vi "Finish.vi"   [LabVIEW 2016]
doc: "This VI is called just before exiting. It is expected to close I/O refnum, save collected data, etc."
uses:
  <vilib>/Rock Robotics/WPI/Utilities/WPI_GetSetVariantRefNum.vi
types:
  T1 = typedef "WPI_EncoderDevRef.ctl" = cluster{"DevStatus":errorcluster, "EncoderIndex":T2, "CounterIndex":T3, "DistancePerCount":dbl, "Decoding Type":T4}
  T2 = typedef "FPGA_EncoderIdx.ctl" = enum8{"Enc 0", "Enc 1", "Enc 2", "Enc 3", "Enc 4", "Enc 5", "Enc 6", "Enc 7", "Invalid"}
  T3 = typedef "FPGA_CounterCtrSystemIndex.ctl" = enum8{"Ctr 0", "Ctr 1", "Ctr 2", "Ctr 3", "Ctr 4", "Ctr 5", "Ctr 6", "Ctr 7", "Invalid"}
  T4 = typedef "WPI_EncoderType.ctl" = enum16{"1x", "2x", "4x"}
  T5 = typedef "WPI_DigitalOutputDevRef.ctl" = cluster{"DIO Channel":T6, "DevStatus":errorcluster}
  T6 = typedef "FPGA_DIOChannel.ctl" = enum8{"DIO 0", "DIO 1", "DIO 2", "DIO 3", "DIO 4", "DIO 5", "DIO 6", "DIO 7", "DIO 8", "DIO 9", "DIO MXP 0", "DIO MXP 1", "DIO MXP 2", "DIO MXP 3", "DIO MXP 4", "DIO MXP 5", "DIO MXP 6", "DIO MXP 7", "DIO MXP 8", "DIO MXP 9", "DIO MXP 10", "DIO MXP 11", "DIO MXP 12", "DIO MXP 13", "DIO MXP 14", "DIO MXP 15", "SPI Port CS1", "SPI Port CS2", "SPI Port CS3", "SPI Port MISO", "SPI Port MOSI", "Invalid"}
  T7 = typedef "WPI_RobotDriveDevRef.ctl" = cluster{"DevStatus":errorcluster, "Motors[]":T8[], "Square Inputs":bool, "Max Output":dbl}
  T8 = typedef "WPI_MotorControlDeviceRef.ctl" = cluster{"DeviceStatus":errorcluster, "Type":T9, "PWM":cluster{"PWM Channel":T10, "DeadBand":T11}, "CAN":cluster{"Device Number":u8, "SetOutput VI Ref":variant, "GetOutput VI Ref":variant, "Enable VI Ref":variant, "Disable VI Ref":variant, "Data":variant}, "Invert":bool}
  T9 = typedef "WPI_MotorControlType.ctl" = enum16{"PWM", "CAN"}
  T10 = typedef "FPGA_DIOPWMChannel.ctl" = enum8{"PWM 0", "PWM 1", "PWM 2", "PWM 3", "PWM 4", "PWM 5", "PWM 6", "PWM 7", "PWM 8", "PWM 9", "PWM MXP 0", "PWM MXP 1", "PWM MXP 2", "PWM MXP 3", "PWM MXP 4", "PWM MXP 5", "PWM MXP 6", "PWM MXP 7", "PWM MXP 8", "PWM MXP 9", "Invalid"}
  T11 = typedef "WPI_PWMDeadband.ctl" = cluster{"Name":string, "maxPositivePwm":i32, "minPositivePwm":i32, "centerPwm":i32, "maxNegativePwm":i32, "minNegativePwm":i32, "angularRange":u16}
  T12 = typedef "WPI_JoystickDevRef.ctl" = cluster{"Device":T13}
  T13 = typedef "WPI_JoystickDeviceEnum.ctl" = enum16{"USB 0", "USB 1", "USB 2", "USB 3", "USB 4", "USB 5"}
  T14 = typedef "WPI_SolenoidDevRef.ctl" = cluster{"DevStatus":errorcluster, "Pneumatics Control Module":u8, "Forward Solenoid Channel":T15, "Reverse Solenoid Channel":T15}
  T15 = typedef "WPI_SolenoidChannel.ctl" = enum8{"Solenoid 0", "Solenoid 1", "Solenoid 2", "Solenoid 3", "Solenoid 4", "Solenoid 5", "Solenoid 6", "Solenoid 7", "Invalid"}
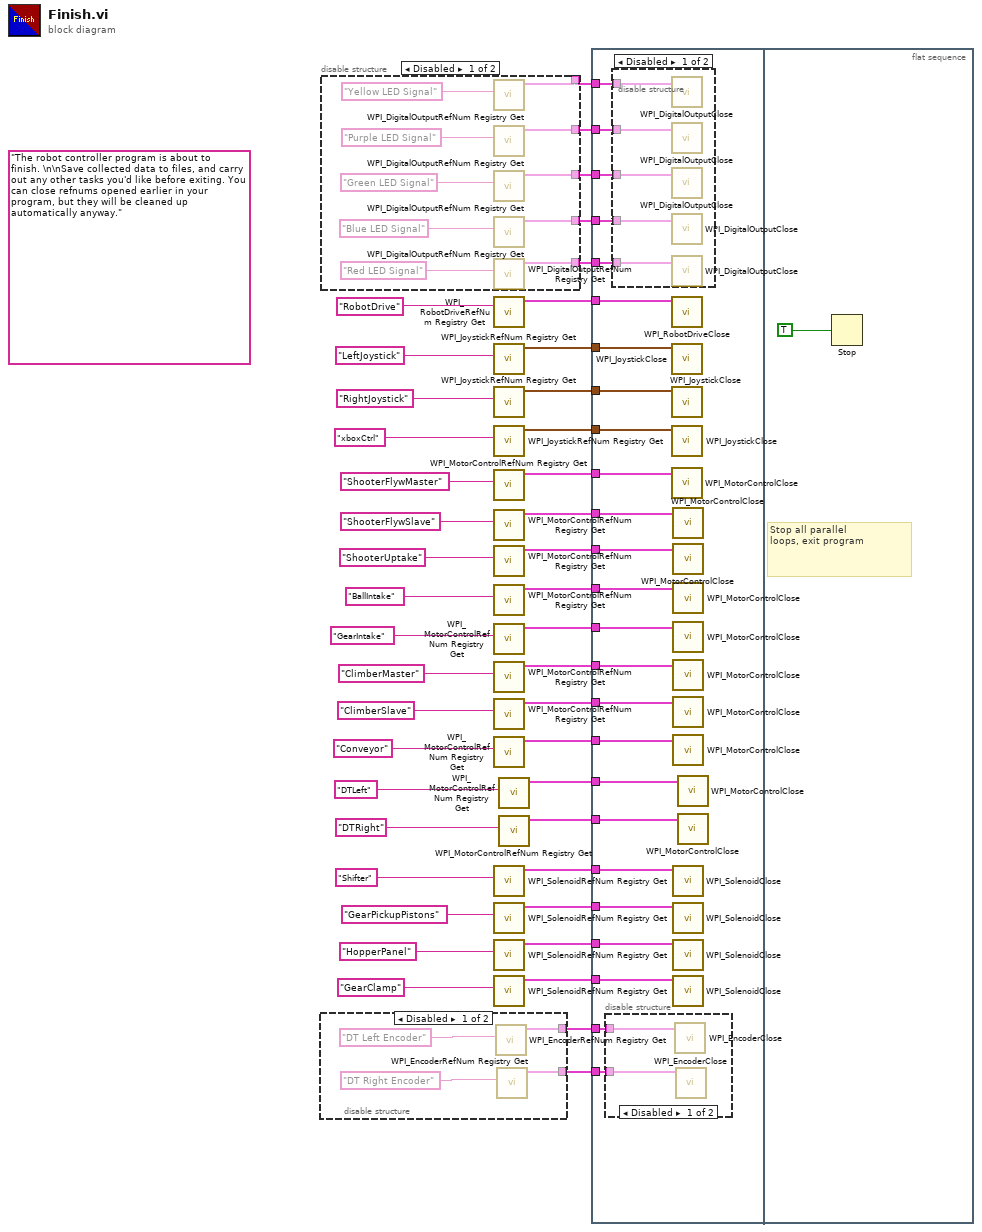
[diagram p0: block diagram]
diagram:
  (unwired) "The robot controller program is about to finish. \n\nSave collected data to files, and carry out any other tasks you'd like before exiting. You can close refnums opened earlier in your program, but they will be cleaned up automatically anyway."
  n1 = disable-structure shown="Disabled" {
    disable-tunnel: [w45 _] -> w6
    disable-tunnel: [w44 _] -> w5
    frame Disabled {
      n2 = call <vilib>:"WPI_EncoderRefNum Registry Get.vi"("refnum name"="DT Left Encoder") -> ("EncoderDevRef"=w45:T1)  [unwired: 9 in, 1 out]
      n3 = call <vilib>:"WPI_EncoderRefNum Registry Get.vi"("refnum name"="DT Right Encoder") -> ("EncoderDevRef"=w44:T1)  [unwired: 9 in, 1 out]
    }
    frame Enabled {
    }
  }
  n4 = disable-structure shown="Disabled" {
    disable-tunnel: [w57 _] -> w11
    disable-tunnel: [w56 _] -> w10
    disable-tunnel: [w55 _] -> w9
    disable-tunnel: [w54 _] -> w8
    disable-tunnel: [w53 _] -> w7
    frame Disabled {
      n5 = call <vilib>:"WPI_DigitalOutputRefNum Registry Get.vi"("refnum name"="Yellow LED Signal") -> ("DigitalOutputDevRef"=w53:T5)  [unwired: 9 in, 1 out]
      n6 = call <vilib>:"WPI_DigitalOutputRefNum Registry Get.vi"("refnum name"="Purple LED Signal") -> ("DigitalOutputDevRef"=w54:T5)  [unwired: 9 in, 1 out]
      n7 = call <vilib>:"WPI_DigitalOutputRefNum Registry Get.vi"("refnum name"="Green LED Signal") -> ("DigitalOutputDevRef"=w55:T5)  [unwired: 9 in, 1 out]
      n8 = call <vilib>:"WPI_DigitalOutputRefNum Registry Get.vi"("refnum name"="Blue LED Signal") -> ("DigitalOutputDevRef"=w56:T5)  [unwired: 9 in, 1 out]
      n9 = call <vilib>:"WPI_DigitalOutputRefNum Registry Get.vi"("refnum name"="Red LED Signal") -> ("DigitalOutputDevRef"=w57:T5)  [unwired: 9 in, 1 out]
    }
    frame Enabled {
    }
  }
  n10 = call <vilib>:"WPI_RobotDriveRefNum Registry Get.vi"("refnum name"="RobotDrive") -> ("RobotDriveDevRef"=w41:T7)  [unwired: 1 in, 9 out]
  n11 = call <vilib>:"WPI_JoystickRefNum Registry Get.vi"("refnum name"="LeftJoystick") -> ("JoystickDevRef"=w40:T12)  [unwired: 1 in, 9 out]
  n12 = call <vilib>:"WPI_JoystickRefNum Registry Get.vi"("refnum name"="RightJoystick") -> ("JoystickDevRef"=w39:T12)  [unwired: 1 in, 9 out]
  n13 = call <vilib>:"WPI_JoystickRefNum Registry Get.vi"("refnum name"="xboxCtrl") -> ("JoystickDevRef"=w36:T12)  [unwired: 1 in, 9 out]
  n14 = call <vilib>:"WPI_MotorControlRefNum Registry Get.vi"("refnum name"="ShooterFlywMaster") -> ("MotorControlDevRef"=w35:T8)  [unwired: 9 in, 1 out]
  n15 = call <vilib>:"WPI_MotorControlRefNum Registry Get.vi"("refnum name"="ShooterFlywSlave") -> ("MotorControlDevRef"=w32:T8)  [unwired: 9 in, 1 out]
  n16 = call <vilib>:"WPI_MotorControlRefNum Registry Get.vi"("refnum name"="ShooterUptake") -> ("MotorControlDevRef"=w31:T8)  [unwired: 9 in, 1 out]
  n17 = call <vilib>:"WPI_MotorControlRefNum Registry Get.vi"("refnum name"="BallIntake") -> ("MotorControlDevRef"=w28:T8)  [unwired: 9 in, 1 out]
  n18 = call <vilib>:"WPI_MotorControlRefNum Registry Get.vi"("refnum name"="GearIntake") -> ("MotorControlDevRef"=w27:T8)  [unwired: 9 in, 1 out]
  n19 = call <vilib>:"WPI_MotorControlRefNum Registry Get.vi"("refnum name"="ClimberMaster") -> ("MotorControlDevRef"=w24:T8)  [unwired: 9 in, 1 out]
  n20 = call <vilib>:"WPI_MotorControlRefNum Registry Get.vi"("refnum name"="ClimberSlave") -> ("MotorControlDevRef"=w23:T8)  [unwired: 9 in, 1 out]
  n21 = call <vilib>:"WPI_MotorControlRefNum Registry Get.vi"("refnum name"="Conveyor") -> ("MotorControlDevRef"=w20:T8)  [unwired: 9 in, 1 out]
  n22 = call <vilib>:"WPI_SolenoidRefNum Registry Get.vi"("refnum name"="Shifter") -> ("SolenoidDevRef"=w19:T14)  [unwired: 9 in, 1 out]
  n23 = call <vilib>:"WPI_SolenoidRefNum Registry Get.vi"("refnum name"="GearPickupPistons") -> ("SolenoidDevRef"=w16:T14)  [unwired: 9 in, 1 out]
  n24 = call <vilib>:"WPI_SolenoidRefNum Registry Get.vi"("refnum name"="HopperPanel") -> ("SolenoidDevRef"=w15:T14)  [unwired: 9 in, 1 out]
  n25 = call <vilib>:"WPI_SolenoidRefNum Registry Get.vi"("refnum name"="GearClamp") -> ("SolenoidDevRef"=w12:T14)  [unwired: 9 in, 1 out]
  n26 = call <vilib>:"WPI_MotorControlRefNum Registry Get.vi"("refnum name"="DTLeft") -> ("MotorControlDevRef"=w1:T8)  [unwired: 9 in, 1 out]
  n27 = call <vilib>:"WPI_MotorControlRefNum Registry Get.vi"("refnum name"="DTRight") -> ("MotorControlDevRef"=w4:T8)  [unwired: 9 in, 1 out]
  n28 = flat-sequence {
    tunnel: w41 -> [w82]
    tunnel: w40 -> [w81]
    tunnel: w39 -> [w80]
    tunnel: w36 -> [w79]
    tunnel: w35 -> [w78]
    tunnel: w32 -> [w77]
    tunnel: w31 -> [w76]
    tunnel: w28 -> [w75]
    tunnel: w27 -> [w74]
    tunnel: w24 -> [w73]
    tunnel: w23 -> [w72]
    tunnel: w20 -> [w71]
    tunnel: w19 -> [w70]
    tunnel: w16 -> [w69]
    tunnel: w15 -> [w68]
    tunnel: w12 -> [w67]
    tunnel: w11 -> [w66]
    tunnel: w10 -> [w65]
    tunnel: w9 -> [w64]
    tunnel: w8 -> [w63]
    tunnel: w7 -> [w62]
    tunnel: w6 -> [w61]
    tunnel: w5 -> [w60]
    tunnel: w1 -> [w58]
    tunnel: w4 -> [w59]
    frame #0 {
      n29 = disable-structure shown="Disabled" {
        disable-tunnel: w61 -> [w89 _]
        disable-tunnel: w60 -> [w88 _]
        frame Disabled {
          n30 = call <vilib>:"WPI_EncoderClose.vi"("EncoderDevRef"=w89) -> ()  [unwired: 10 in, 1 out]
          n31 = call <vilib>:"WPI_EncoderClose.vi"("EncoderDevRef"=w88) -> ()  [unwired: 10 in, 1 out]
        }
        frame Enabled {
        }
      }
      n32 = disable-structure shown="Disabled" {
        disable-tunnel: w66 -> [w87 _]
        disable-tunnel: w65 -> [w86 _]
        disable-tunnel: w64 -> [w85 _]
        disable-tunnel: w63 -> [w84 _]
        disable-tunnel: w62 -> [w83 _]
        frame Disabled {
          n33 = call <vilib>:"WPI_DigitalOutputClose.vi"("DigitalOutputDevRef"=w83) -> ()  [unwired: 10 in, 1 out]
          n34 = call <vilib>:"WPI_DigitalOutputClose.vi"("DigitalOutputDevRef"=w84) -> ()  [unwired: 10 in, 1 out]
          n35 = call <vilib>:"WPI_DigitalOutputClose.vi"("DigitalOutputDevRef"=w85) -> ()  [unwired: 10 in, 1 out]
          n36 = call <vilib>:"WPI_DigitalOutputClose.vi"("DigitalOutputDevRef"=w86) -> ()  [unwired: 10 in, 1 out]
          n37 = call <vilib>:"WPI_DigitalOutputClose.vi"("DigitalOutputDevRef"=w87) -> ()  [unwired: 10 in, 1 out]
        }
        frame Enabled {
        }
      }
      n38 = call <vilib>:"WPI_RobotDriveClose.vi"("RobotDriveDevRef"=w82) -> ()  [unwired: 1 in, 10 out]
      n39 = call <vilib>:"WPI_JoystickClose.vi"("JoystickDevRef"=w81) -> ()  [unwired: 11 out]
      n40 = call <vilib>:"WPI_JoystickClose.vi"("JoystickDevRef"=w80) -> ()  [unwired: 11 out]
      n41 = call <vilib>:"WPI_JoystickClose.vi"("JoystickDevRef"=w79) -> ()  [unwired: 11 out]
      n42 = call <vilib>:"WPI_MotorControlClose.vi"("MotorControlDevRef"=w78) -> ()  [unwired: 10 in, 1 out]
      n43 = call <vilib>:"WPI_MotorControlClose.vi"("MotorControlDevRef"=w77) -> ()  [unwired: 10 in, 1 out]
      n44 = call <vilib>:"WPI_MotorControlClose.vi"("MotorControlDevRef"=w76) -> ()  [unwired: 10 in, 1 out]
      n45 = call <vilib>:"WPI_MotorControlClose.vi"("MotorControlDevRef"=w75) -> ()  [unwired: 10 in, 1 out]
      n46 = call <vilib>:"WPI_MotorControlClose.vi"("MotorControlDevRef"=w74) -> ()  [unwired: 10 in, 1 out]
      n47 = call <vilib>:"WPI_MotorControlClose.vi"("MotorControlDevRef"=w73) -> ()  [unwired: 10 in, 1 out]
      n48 = call <vilib>:"WPI_MotorControlClose.vi"("MotorControlDevRef"=w72) -> ()  [unwired: 10 in, 1 out]
      n49 = call <vilib>:"WPI_MotorControlClose.vi"("MotorControlDevRef"=w71) -> ()  [unwired: 10 in, 1 out]
      n50 = call <vilib>:"WPI_SolenoidClose.vi"("SolenoidDevRef"=w70) -> ()  [unwired: 10 in, 1 out]
      n51 = call <vilib>:"WPI_SolenoidClose.vi"("SolenoidDevRef"=w69) -> ()  [unwired: 10 in, 1 out]
      n52 = call <vilib>:"WPI_SolenoidClose.vi"("SolenoidDevRef"=w68) -> ()  [unwired: 10 in, 1 out]
      n53 = call <vilib>:"WPI_SolenoidClose.vi"("SolenoidDevRef"=w67) -> ()  [unwired: 10 in, 1 out]
      n54 = call <vilib>:"WPI_MotorControlClose.vi"("MotorControlDevRef"=w58) -> ()  [unwired: 10 in, 1 out]
      n55 = call <vilib>:"WPI_MotorControlClose.vi"("MotorControlDevRef"=w59) -> ()  [unwired: 10 in, 1 out]
    }
    frame #1 {
      # "Stop all parallel\nloops, exit program"
      n56 = Stop(stop? (T)=TRUE ("Quit")) -> ()
    }
  }
